vi "Write NET_HttpClient.vi"(8 "error in (no error)":errorcluster, 10 "NET_HttpClient":refnum<k24>, 11 "LabVIEWHTTPClient_NET in":refnum<class "HttpClient_NET.lvclass">) -> (0 "error out":errorcluster, 3 "LabVIEWHTTPClient_NET out":refnum<class "HttpClient_NET.lvclass">)   [LabVIEW 2018, in "HttpClient_NET.lvlib" / "HttpClient_NET.lvclass"]
doc: "<b> </b> <b> </b>\nHttpClient_NET\nJustin Young - Viviota\nCopyright (c) 2021\nLicense: BSD"
uses:
  HttpClient_NET.lvclass
  System.Net.Http
  HttpClient_NET.lvclass/HttpClient_NET.ctl
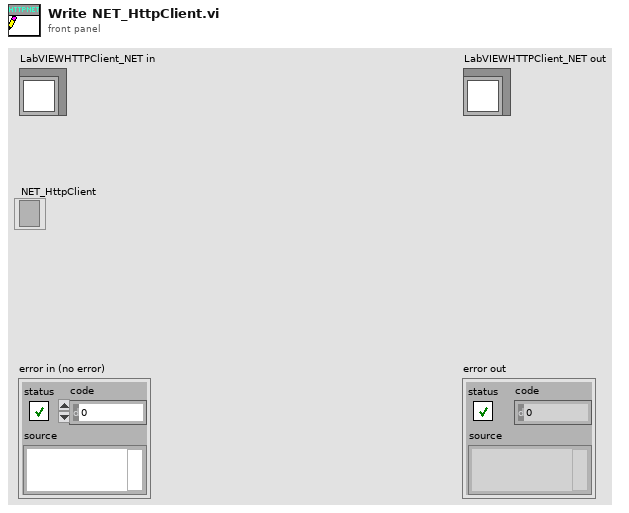
[diagram p1: front panel]
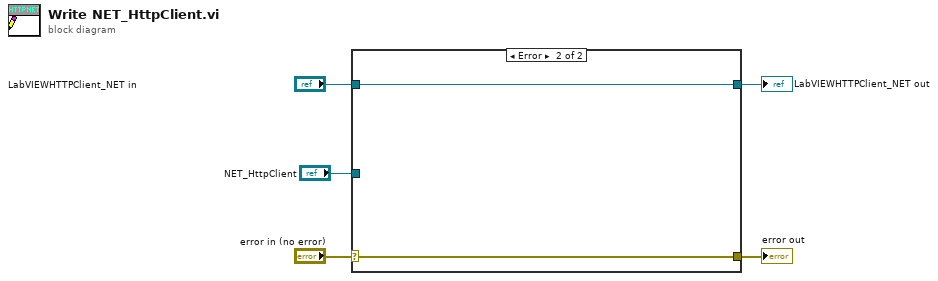
[diagram p0: block diagram]
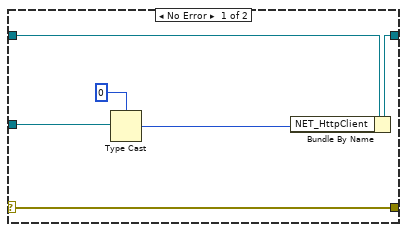
[diagram p2: hidden frame]
diagram:
  n1 = case shown="Error" "error in (no error)" {
    selector: "error in (no error)" -> [w11 w12]
    tunnel: [w11 w12] -> w4
    tunnel: [w9 w13] -> w2
    tunnel: "LabVIEWHTTPClient_NET in" -> [w10 w13]
    tunnel: "NET_HttpClient" -> [w8 _]
    frame No Error {
      n2 = Type Cast(type=i64 0 ("NET_HttpClient"), x=w8) -> (*(type *) &x=w6:i64)
      n3 = Bundle By Name(cluster=w10, "NET_HttpClient"=w6) -> (w9:refnum<class "HttpClient_NET.lvclass">)
    }
    frame Error {
    }
  }
  "error out" <- w4
  "LabVIEWHTTPClient_NET out" <- w2
